vi "Update JSON Config Req.vi"(8 "error in (no error)":errorcluster, 10 "ConfigRequest":T1={"SMUResourceName"="SMU1", "SMUChannels"="0:1", "SMUSourceMode"=1022, "SMUOutputFunction"=1008, "SMUSourceTransientResponse"=1040, "SMUCurrent"=2.0, "SMUCurrentLevelRange"=2.0, "SMUMeasurementSense"=1009, "SMUMeasurementApertureTime"=0.011, "SMUSourceAdvancedSourceDelay"=0.000101, "SMUVoltage"=7.0, "SMUSourceAdvancedSequenceLoopCount"=701, "SMUMeasurementAdvancedDCNoiseRejection"=1045, "SMUSequenceName"="YourSequence", "ScanList"="", "DMMResourceName"="DMM1", "DMMFunction"=1, "DMMResolution"=0.2, "DMMRange"=0.2, "DMMSampleCount"=1, "DMMApertureTimeUnit"=1, "DMMApertureTime"=0.011, "DMMNumberOfAverages"=2, "DMMAutoZero"=1, "DMMADCCalibration"=1, "DMMSettleTime"=0.0002, "DMMControlAction"=1, "DMMVoltageFaultUpperLimit"=5.1e-05, "ApplicationNumberOfWeldChannels"=8}, 11 "JSON Configuration File (.json)":path=path "C:/Users/chericks/Desktop/JSONfun/jsonbefore.json") -> (0 "error out":errorcluster)   [LabVIEW 2019]
uses:
  JSONCluster.ctl
  labview-grpc-query-server/VIs/MeasurementServer_ConfigRequest.ctl
  labview-grpc-query-server/VIs/labview-grpc-measurement-server.lvlib
panel:
  out "File Contents":string="{\n    \"SMUResourceName\": \"SMU\",\n    \"SMUChannels\": \"0\",\n\t\"SMUSourceMode\": 1021,\n\t\"SMUOutputFunction\": 1007,\n    \"SMUSourceTransientResponse\": 1039,\n    \"SMUCurrent\": 1.0,\n    \"SMUCurrentLevelRange\": 1.0,\n    \"SMUMeasurementSense\": 1008,\n    \"SMUMeasurementApertureTime\": 0.010,\n    \"SMUSourceAdvancedSourceDelay\": 0.000100,\n    \"SMUVoltage\": 6,\n    \"SMUSourceAdvancedSequenceLoopCount\": 700,\n    \"SMUMeasurementAdvancedDCNoiseRejection\": 1044,\n\t\"SMUSequenceName\": \"MySequence\",\n\t\"SMUStep1_Source_DCCurrent_CurrentLevel\": 1150009,\n\t\"SMUStep2_Measurement_ApertureTime\": 1150058,\n\t\"SMUStep3_Source_Advanced_SourceDelay\": 1150051,\n\t\"SMUSequenceNumberOfSteps\": 3,\n\t\t\n\t\"Switch1ResourceName\": \"2526_1\",\n\t\"Switch1Topology\": \"2526/2-Wire 79x1 Mux\",\n\t\"Switch1ScanList\": \"ch70:76->com\",\n\t\n\t\"Switch2ResourceName\": \"SwitchBlock1Dev1\",\n\t\"Switch2Topology\": \"Configured Topology\",\n\t\"Switch2ScanList\": \"[c2->card1r2->c26], [c3->card1r3->c27]; [c6->card1r2->c26], [c7->card1r3->c27]; [c10->card1r2->c26], [c11->card1r3->c27]; [c14->card1r2->c26], [c15->card1r3->c27]; [c18->card1r2->c26], [c19->card1r3->c27]; [c22->card1r2->c26], [c23->card1r3->c27]; [c30->card1r2->c26], [c31->card1r3->c27];\",\n\t\n\t\"DMMResourceName\": \"DMM\",\n\t\"DMMFunction\": 0,\n\t\"DMMResolution\": 0.1,\n\t\"DMMRange\": 0.1,\n\t\"DMMSampleCount\": 0,\n\t\"DMMApertureTimeUnit\": 0,\n\t\"DMMApertureTime\": 0.010,\n\t\"DMMNumberOfAverages\": 1,\n\t\"DMMAutoZero\": 0,\n\t\"DMMADCCalibration\": 0,\n\t\"DMMSettleTime\": 0.0001,\n\t\"DMMControlAction\": 0,\n\t\"DMMVoltageFaultUpperLimit\": 0.000050,\n\t\n\t\"ApplicationNumberOfWeldChannels\": 7\n}"
  out "JSONCluster":T2={"SMUResourceName"="SMU", "SMUChannels"="0", "SMUSourceMode"=1021, "SMUOutputFunction"=1007, "SMUSourceTransientResponse"=1039, "SMUCurrent"=1.0, "SMUCurrentLevelRange"=1.0, "SMUMeasurementSense"=1008, "SMUMeasurementApertureTime"=0.01, "SMUSourceAdvancedSourceDelay"=0.0001, "SMUVoltage"=6.0, "SMUSourceAdvancedSequenceLoopCount"=700, "SMUMeasurementAdvancedDCNoiseRejection"=1044, "SMUSequenceName"="MySequence", "SMUStep1_Source_DCCurrent_CurrentLevel"=1150009, "SMUStep2_Measurement_ApertureTime"=1150058, "SMUStep3_Source_Advanced_SourceDelay"=1150051, "SMUSequenceNumberOfSteps"=3, "Switch1ResourceName"="2526_1", "Switch1Topology"="2526/2-Wire 79x1 Mux", "Switch1ScanList"="ch70:76->com", "Switch2ResourceName"="SwitchBlock1Dev1", "Switch2Topology"="Configured Topology", "Switch2ScanList"="[c2->card1r2->c26], [c3->card1r3->c27]; [c6->card1r2->c26], [c7->card1r3->c27]; [c10->card1r2->c26], [c11->card1r3->c27]; [c14->card1r2->c26], [c15->card1r3->c27]; [c18->card1r2->c26], [c19->card1r3->c27]; [c22->card1r2->c26], [c23->card1r3->c27]; [c30->card1r2->c26], [c31->card1r3->c27];", "DMMResourceName"="DMM", "DMMFunction"=0, "DMMResolution"=0.1, "DMMRange"=0.1, "DMMSampleCount"=0, "DMMApertureTimeUnit"=0, "DMMApertureTime"=0.01, "DMMNumberOfAverages"=1, "DMMAutoZero"=0, "DMMADCCalibration"=0, "DMMSettleTime"=0.0001, "DMMControlAction"=0, "DMMVoltageFaultUpperLimit"=5e-05, "ApplicationNumberOfWeldChannels"=7}
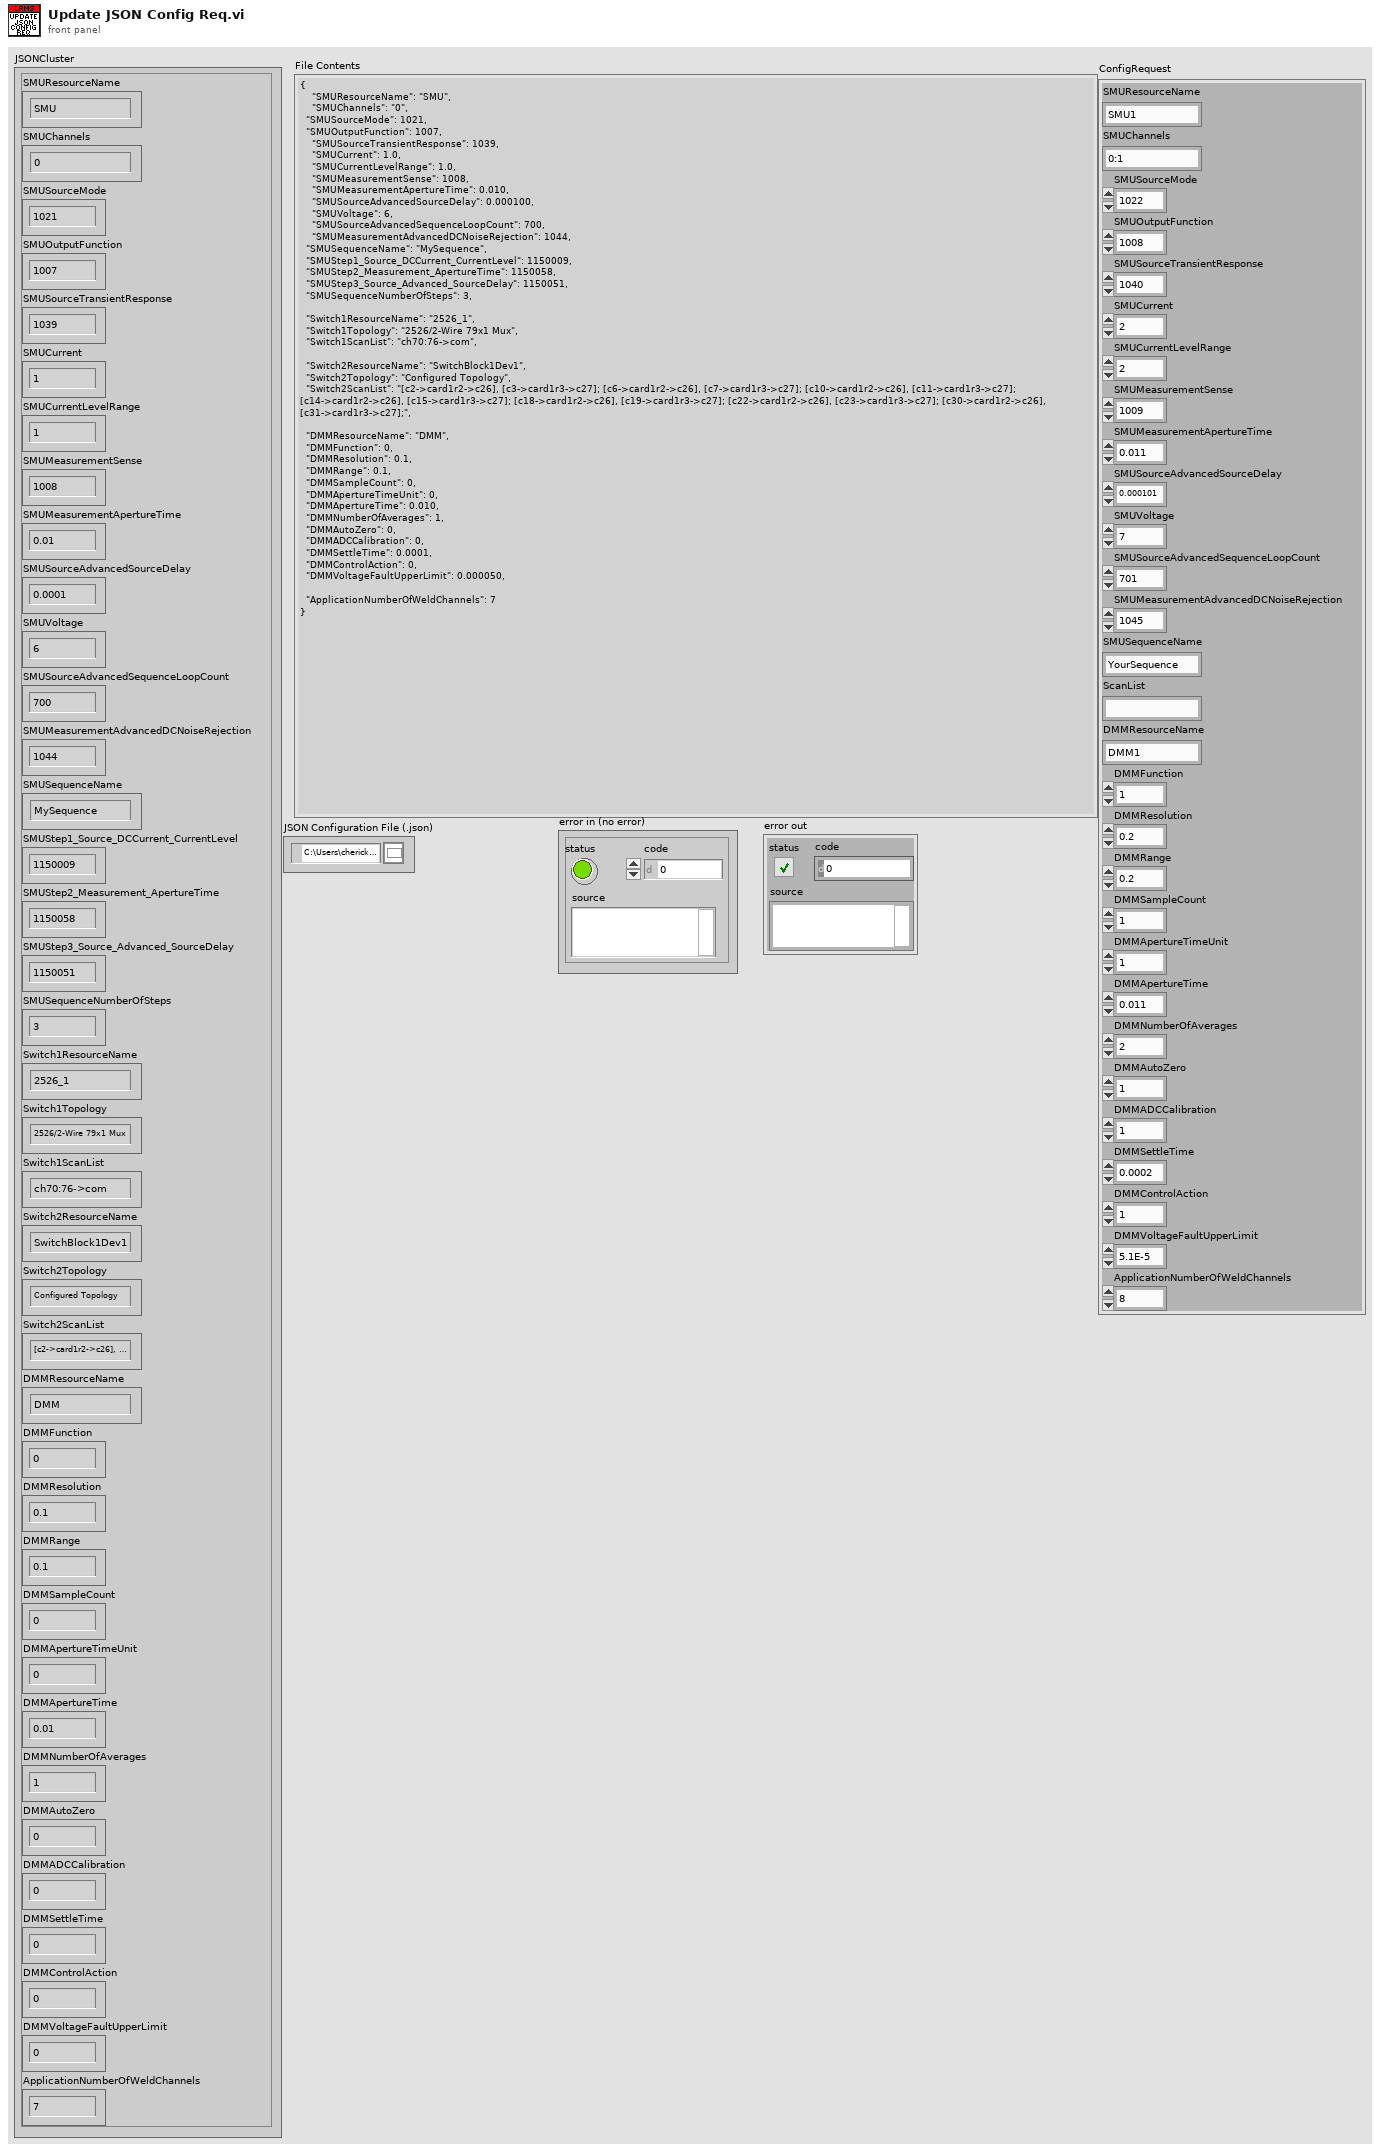
[diagram p1: front panel]
types:
  T1 = typedef "labview-grpc-measurement-server.lvlib/MeasurementServer_ConfigRequest.ctl" = cluster{"SMUResourceName":string, "SMUChannels":string, "SMUSourceMode":i32, "SMUOutputFunction":i32, "SMUSourceTransientResponse":i32, "SMUCurrent":sgl, "SMUCurrentLevelRange":sgl, "SMUMeasurementSense":i32, "SMUMeasurementApertureTime":sgl, "SMUSourceAdvancedSourceDelay":sgl, "SMUVoltage":sgl, "SMUSourceAdvancedSequenceLoopCount":i32, "SMUMeasurementAdvancedDCNoiseRejection":i32, "SMUSequenceName":string, "ScanList":string, "DMMResourceName":string, "DMMFunction":i32, "DMMResolution":sgl, "DMMRange":sgl, "DMMSampleCount":i32, "DMMApertureTimeUnit":i32, "DMMApertureTime":sgl, "DMMNumberOfAverages":i32, "DMMAutoZero":i32, "DMMADCCalibration":i32, "DMMSettleTime":sgl, "DMMControlAction":i32, "DMMVoltageFaultUpperLimit":sgl, "ApplicationNumberOfWeldChannels":i32}
  T2 = typedef "JSONCluster.ctl" = cluster{"SMUResourceName":string, "SMUChannels":string, "SMUSourceMode":i32, "SMUOutputFunction":i32, "SMUSourceTransientResponse":i32, "SMUCurrent":dbl, "SMUCurrentLevelRange":dbl, "SMUMeasurementSense":i32, "SMUMeasurementApertureTime":dbl, "SMUSourceAdvancedSourceDelay":dbl, "SMUVoltage":dbl, "SMUSourceAdvancedSequenceLoopCount":i32, "SMUMeasurementAdvancedDCNoiseRejection":i32, "SMUSequenceName":string, "SMUStep1_Source_DCCurrent_CurrentLevel":i32, "SMUStep2_Measurement_ApertureTime":i32, "SMUStep3_Source_Advanced_SourceDelay":i32, "SMUSequenceNumberOfSteps":i32, "Switch1ResourceName":string, "Switch1Topology":string, "Switch1ScanList":string, "Switch2ResourceName":string, "Switch2Topology":string, "Switch2ScanList":string, "DMMResourceName":string, "DMMFunction":i32, "DMMResolution":dbl, "DMMRange":dbl, "DMMSampleCount":i32, "DMMApertureTimeUnit":i32, "DMMApertureTime":dbl, "DMMNumberOfAverages":i32, "DMMAutoZero":i32, "DMMADCCalibration":i32, "DMMSettleTime":dbl, "DMMControlAction":i32, "DMMVoltageFaultUpperLimit":dbl, "ApplicationNumberOfWeldChannels":i32}
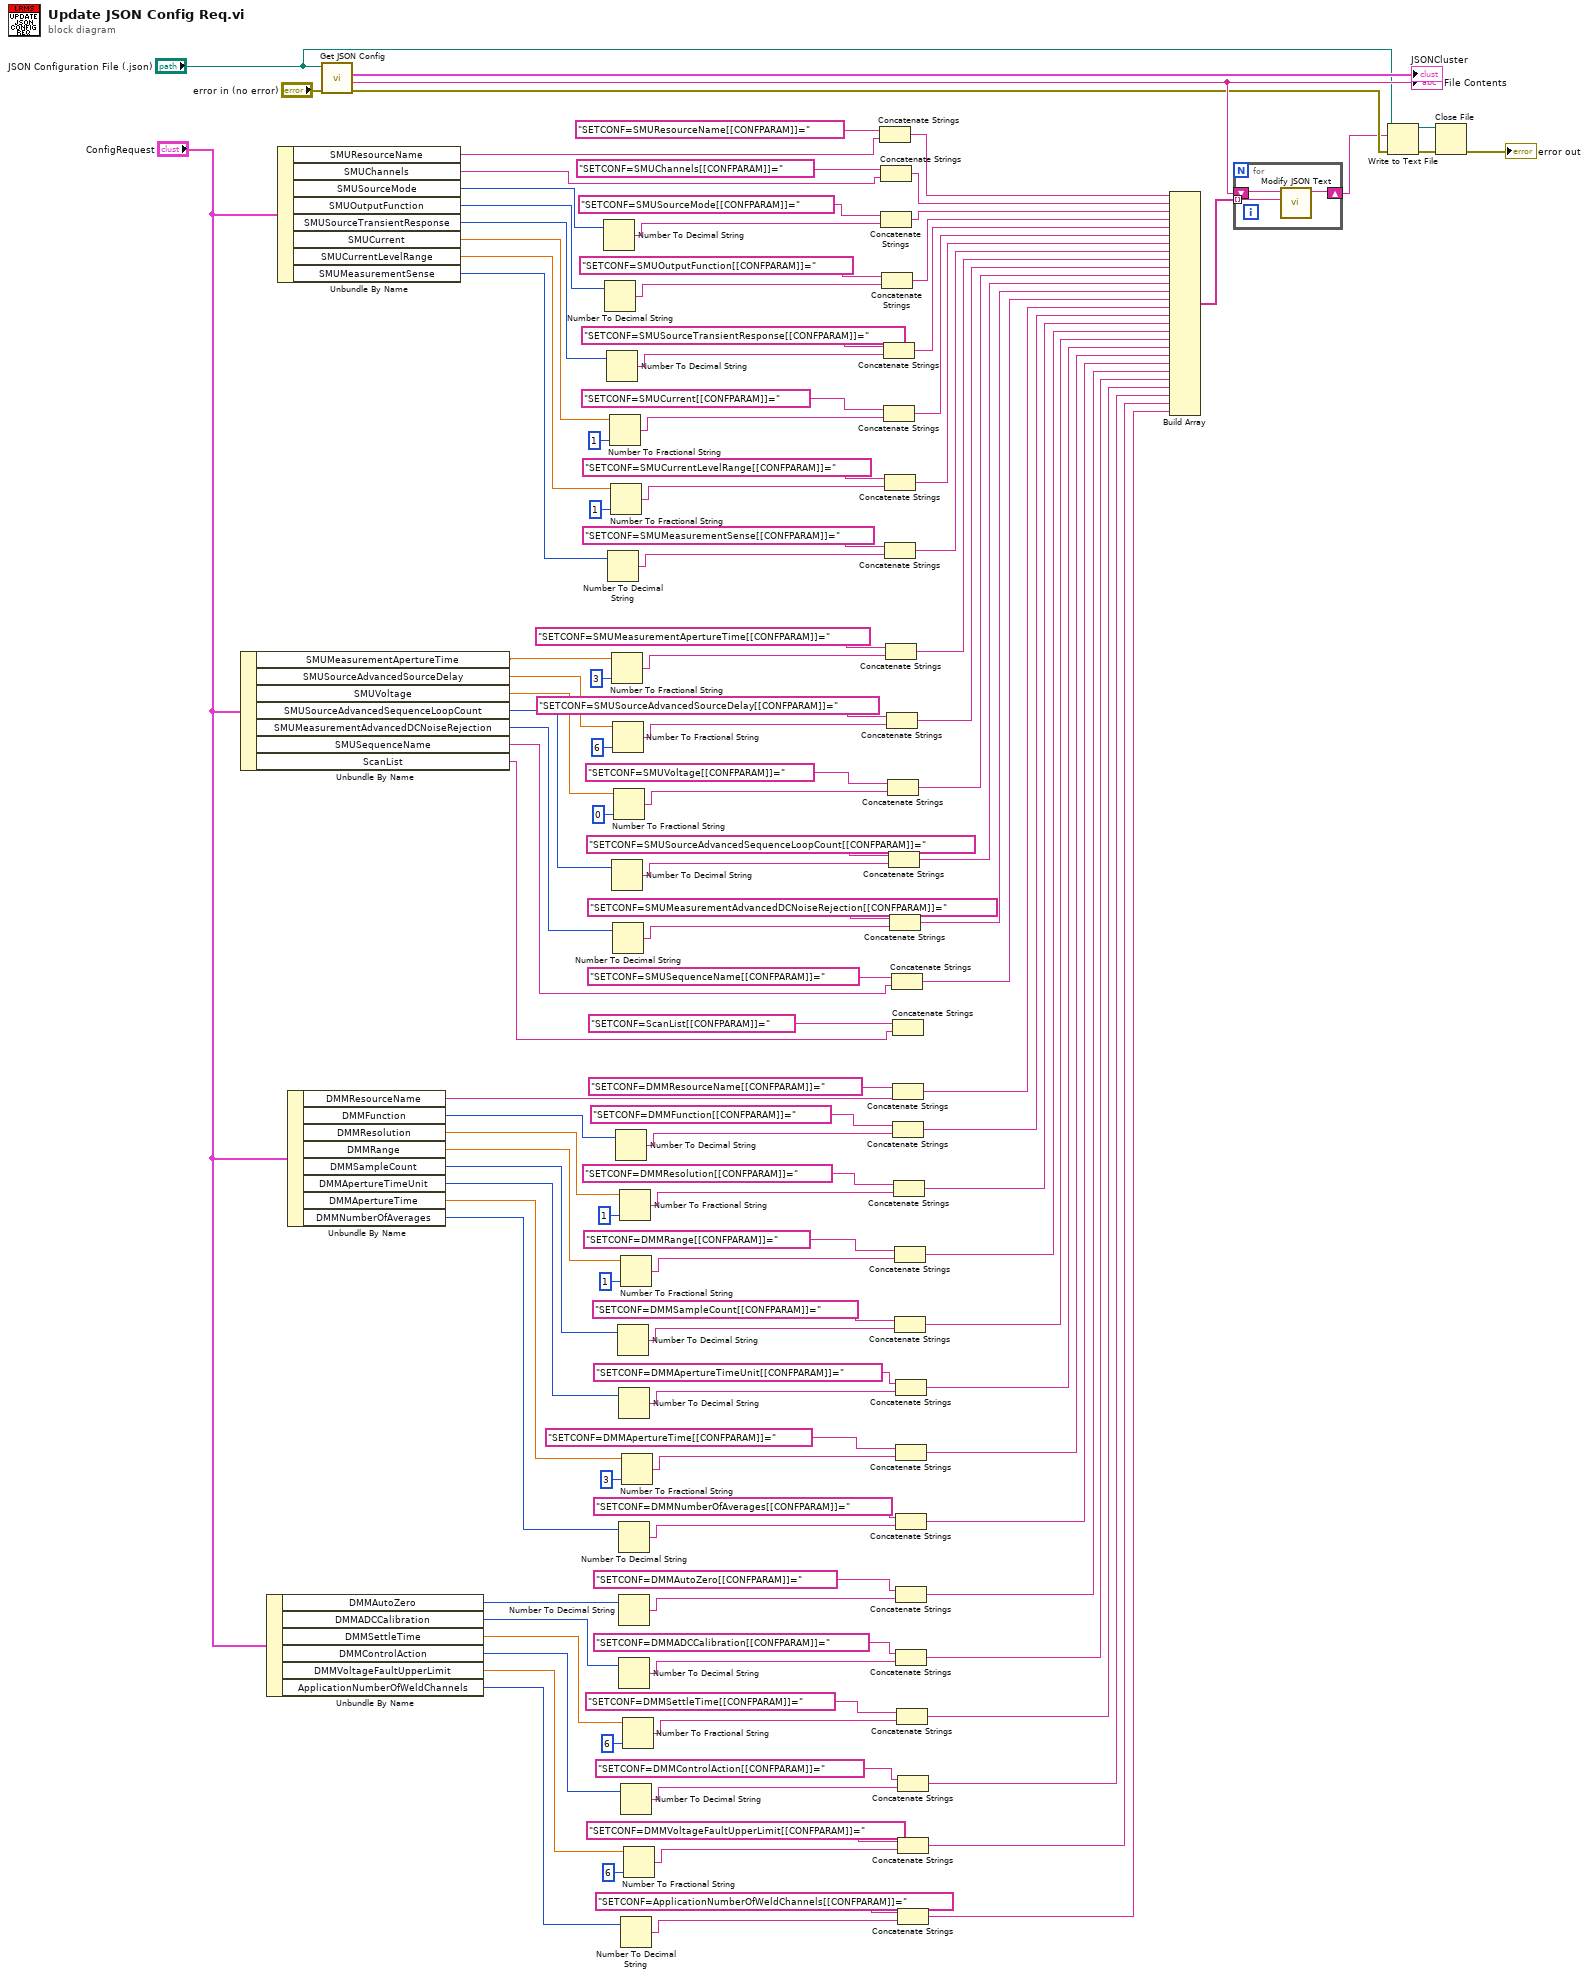
[diagram p0: block diagram]
diagram:
  n1 = Unbundle By Name("ConfigRequest") -> ("SMUMeasurementApertureTime"=w85:sgl, "SMUSourceAdvancedSourceDelay"=w84:sgl, "SMUVoltage"=w78:sgl, "SMUSourceAdvancedSequenceLoopCount"=w74:i32, "SMUMeasurementAdvancedDCNoiseRejection"=w70:i32, "SMUSequenceName"=w67:string, "ScanList"=w64:string)
  n2 = Unbundle By Name("ConfigRequest") -> ("DMMAutoZero"=w26:i32, "DMMADCCalibration"=w22:i32, "DMMSettleTime"=w18:sgl, "DMMControlAction"=w13:i32, "DMMVoltageFaultUpperLimit"=w8:sgl, "ApplicationNumberOfWeldChannels"=w4:i32)
  n3 = Unbundle By Name("ConfigRequest") -> ("SMUResourceName"=w129:string, "SMUChannels"=w126:string, "SMUSourceMode"=w117:i32, "SMUOutputFunction"=w111:i32, "SMUSourceTransientResponse"=w107:i32, "SMUCurrent"=w104:sgl, "SMUCurrentLevelRange"=w97:sgl, "SMUMeasurementSense"=w93:i32)
  n4 = Unbundle By Name("ConfigRequest") -> ("DMMResourceName"=w62:string, "DMMFunction"=w58:i32, "DMMResolution"=w53:sgl, "DMMRange"=w49:sgl, "DMMSampleCount"=w44:i32, "DMMApertureTimeUnit"=w41:i32, "DMMApertureTime"=w35:sgl, "DMMNumberOfAverages"=w31:i32)
  n5 = call "Get JSON Config.vi"("error in (no error)"="error in (no error)", "JSON Configuration File (.json)"="JSON Configuration File (.json)") -> ("error out"=w119:errorcluster, "File Contents"=w128:string, "JSONCluster"=→"JSONCluster":T2)  [unwired: 6 in, 1 out]
  "File Contents" <- w128
  n6 = Number To Decimal String(number=w117) -> (decimal integer string=w115:string)  [unwired: 1 in]
  n7 = Number To Decimal String(number=w111) -> (decimal integer string=w112:string)  [unwired: 1 in]
  n8 = Number To Decimal String(number=w107) -> (decimal integer string=w108:string)  [unwired: 1 in]
  n9 = Number To Decimal String(number=w93) -> (decimal integer string=w94:string)  [unwired: 1 in]
  n10 = Number To Fractional String(number=w104, precision (6)=i16 1) -> (F-format string=w103:string)  [unwired: 2 in]
  n11 = Number To Fractional String(number=w97, precision (6)=i16 1) -> (F-format string=w99:string)  [unwired: 2 in]
  n12 = Number To Fractional String(number=w85, precision (6)=i16 3) -> (F-format string=w90:string)  [unwired: 2 in]
  n13 = Number To Decimal String(number=w74) -> (decimal integer string=w75:string)  [unwired: 1 in]
  n14 = Number To Fractional String(number=w84, precision (6)=i16 6) -> (F-format string=w87:string)  [unwired: 2 in]
  n15 = Number To Decimal String(number=w70) -> (decimal integer string=w71:string)  [unwired: 1 in]
  n16 = Number To Fractional String(number=w78, precision (6)=i16 0) -> (F-format string=w80:string)  [unwired: 2 in]
  n17 = Number To Decimal String(number=w58) -> (decimal integer string=w59:string)  [unwired: 1 in]
  n18 = Number To Decimal String(number=w44) -> (decimal integer string=w45:string)  [unwired: 1 in]
  n19 = Number To Decimal String(number=w41) -> (decimal integer string=w42:string)  [unwired: 1 in]
  n20 = Number To Decimal String(number=w31) -> (decimal integer string=w33:string)  [unwired: 1 in]
  n21 = Number To Decimal String(number=w26) -> (decimal integer string=w28:string)  [unwired: 1 in]
  n22 = Number To Decimal String(number=w22) -> (decimal integer string=w24:string)  [unwired: 1 in]
  n23 = Number To Fractional String(number=w53, precision (6)=i16 1) -> (F-format string=w55:string)  [unwired: 2 in]
  n24 = Number To Fractional String(number=w49, precision (6)=i16 1) -> (F-format string=w51:string)  [unwired: 2 in]
  n25 = Number To Decimal String(number=w13) -> (decimal integer string=w15:string)  [unwired: 1 in]
  n26 = Number To Decimal String(number=w4) -> (decimal integer string=w6:string)  [unwired: 1 in]
  n27 = Number To Fractional String(number=w35, precision (6)=i16 3) -> (F-format string=w37:string)  [unwired: 2 in]
  n28 = Number To Fractional String(number=w18, precision (6)=i16 6) -> (F-format string=w20:string)  [unwired: 2 in]
  n29 = Number To Fractional String(number=w8, precision (6)=i16 6) -> (F-format string=w11:string)  [unwired: 2 in]
  n30 = Concatenate Strings("SETCONF=SMUResourceName[[CONFPARAM]]=", w129) -> (w127:string)
  n31 = Concatenate Strings("SETCONF=SMUChannels[[CONFPARAM]]=", w126) -> (w124:string)
  n32 = Concatenate Strings("SETCONF=SMUSourceMode[[CONFPARAM]]=", w115) -> (w114:string)
  n33 = Concatenate Strings("SETCONF=SMUOutputFunction[[CONFPARAM]]=", w112) -> (w110:string)
  n34 = Concatenate Strings("SETCONF=SMUSourceTransientResponse[[CONFPARAM]]=", w108) -> (w106:string)
  n35 = Concatenate Strings("SETCONF=SMUCurrent[[CONFPARAM]]=", w103) -> (w102:string)
  n36 = Concatenate Strings("SETCONF=SMUCurrentLevelRange[[CONFPARAM]]=", w99) -> (w96:string)
  n37 = Concatenate Strings("SETCONF=SMUMeasurementSense[[CONFPARAM]]=", w94) -> (w92:string)
  n38 = Concatenate Strings("SETCONF=SMUMeasurementApertureTime[[CONFPARAM]]=", w90) -> (w83:string)
  n39 = Concatenate Strings("SETCONF=SMUSourceAdvancedSourceDelay[[CONFPARAM]]=", w87) -> (w82:string)
  n40 = Concatenate Strings("SETCONF=SMUVoltage[[CONFPARAM]]=", w80) -> (w77:string)
  n41 = Concatenate Strings("SETCONF=SMUSourceAdvancedSequenceLoopCount[[CONFPARAM]]=", w75) -> (w73:string)
  n42 = Concatenate Strings("SETCONF=SMUMeasurementAdvancedDCNoiseRejection[[CONFPARAM]]=", w71) -> (w69:string)
  n43 = Concatenate Strings("SETCONF=SMUSequenceName[[CONFPARAM]]=", w67) -> (w66:string)
  n44 = Concatenate Strings("SETCONF=ScanList[[CONFPARAM]]=", w64) -> ()  [unwired: 1 out]
  n45 = Concatenate Strings("SETCONF=DMMResourceName[[CONFPARAM]]=", w62) -> (w61:string)
  n46 = Concatenate Strings("SETCONF=DMMFunction[[CONFPARAM]]=", w59) -> (w57:string)
  n47 = Concatenate Strings("SETCONF=DMMResolution[[CONFPARAM]]=", w55) -> (w52:string)
  n48 = Concatenate Strings("SETCONF=DMMRange[[CONFPARAM]]=", w51) -> (w47:string)
  n49 = Concatenate Strings("SETCONF=DMMSampleCount[[CONFPARAM]]=", w45) -> (w43:string)
  n50 = Concatenate Strings("SETCONF=DMMApertureTimeUnit[[CONFPARAM]]=", w42) -> (w39:string)
  n51 = Concatenate Strings("SETCONF=DMMApertureTime[[CONFPARAM]]=", w37) -> (w34:string)
  n52 = Concatenate Strings("SETCONF=DMMNumberOfAverages[[CONFPARAM]]=", w33) -> (w30:string)
  n53 = Concatenate Strings("SETCONF=DMMAutoZero[[CONFPARAM]]=", w28) -> (w25:string)
  n54 = Concatenate Strings("SETCONF=DMMADCCalibration[[CONFPARAM]]=", w24) -> (w21:string)
  n55 = Concatenate Strings("SETCONF=DMMSettleTime[[CONFPARAM]]=", w20) -> (w16:string)
  n56 = Concatenate Strings("SETCONF=DMMControlAction[[CONFPARAM]]=", w15) -> (w12:string)
  n57 = Concatenate Strings("SETCONF=DMMVoltageFaultUpperLimit[[CONFPARAM]]=", w11) -> (w7:string)
  n58 = Concatenate Strings("SETCONF=ApplicationNumberOfWeldChannels[[CONFPARAM]]=", w6) -> (w3:string)
  n59 = Build Array(w127, w124, w114, w110, w106, w102, w96, w92, w83, w82, w77, w73, w69, w66, w61, w57, w52, w47, w43, w39, w34, w30, w25, w21, w16, w12, w7, w3) -> (w123:string[])
  n60 = for {
    tunnel: w123 -> [w134] mode=indexing
    shift-right: [w133] -> w118
    shift-left: w128 -> [w132]
    n61 = call "Modify JSON Text.vi"("Parameter and Value"=w134, "JSONtextin"=w132) -> ("JSONtextout"=w133:string)  [unwired: 9 in]
  }
  n62 = Write to Text File(file (use dialog)="JSON Configuration File (.json)", text=w118, error in=w119) -> (refnum out=w122:refnum<file>, error out=w121:errorcluster)  [unwired: 1 in, 1 out]
  n63 = Close File(refnum=w122, error in=w121) -> (error out=→"error out":errorcluster)  [unwired: 1 out]
